vi "FTW-WebService-GetURI.vi"(8 "error in":errorcluster, 11 "FTW Web Request":refnum<class "FTW-WebService.lvclass">) -> (0 "error out":errorcluster, 2 "RequestURI":string, 3 "FTW Web Request out":refnum<class "FTW-WebService.lvclass">)   [LabVIEW 2014, in "FTW-WebService.lvclass"]
uses:
  FTW-WebService.lvclass
  FTW-WebService.lvclass/FTW-WebService.ctl
panel:
  # "Inputs"
  # "Outputs"
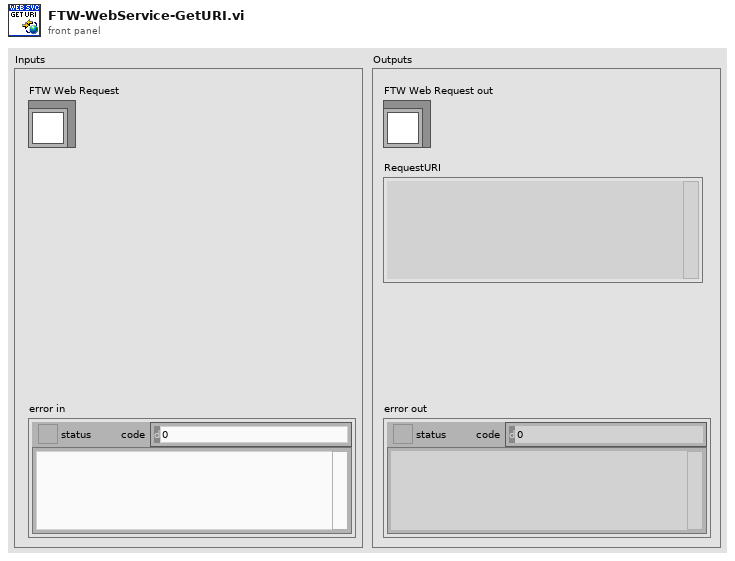
[diagram p1: front panel]
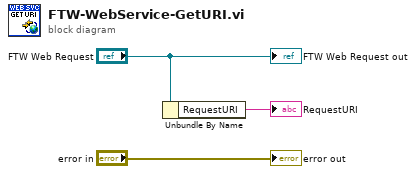
[diagram p0: block diagram]
diagram:
  n1 = Unbundle By Name("FTW Web Request") -> ("RequestURI"=→"RequestURI":string)
  "error out" <- "error in"
  "FTW Web Request out" <- "FTW Web Request"
